vi "Process Data.vi"(7 "AdasLvTemplate in":refnum<class "AdasLvTemplate.lvclass">, 8 "error in":errorcluster, 11 "Node in":refnum<class "AMS Chiller Template.lvclass">) -> (0 "error out":errorcluster, 3 "Node out":refnum<class "AMS Chiller Template.lvclass">, 5 "AdasLvTemplate out":refnum<class "AdasLvTemplate.lvclass">)   [LabVIEW 2023, in "AMS Chiller Template.lvlib" / "AMS Chiller Template.lvclass"]
uses:
  AMS Chiller Template.lvclass
  <vilib>/ADAS Replay HIL/ADAS Plugin Utilities/AdasLvTemplate/AdasLvTemplate.lvclass
  AMS Chiller Template.lvclass/AMS Chiller Template.ctl
  C:/Program Files/National Instruments/AMS plugin/Capabilities/Capabilities/High Level Capabilities/Chiller/Control Mode Read Array.vi
  C:/Program Files/National Instruments/AMS plugin/Capabilities/Capabilities/High Level Capabilities/Chiller/Control Mode Write Array.vi
  C:/Program Files/National Instruments/AMS plugin/Capabilities/Capabilities/High Level Capabilities/Chiller/Output Enable Read Array.vi
  C:/Program Files/National Instruments/AMS plugin/Capabilities/Capabilities/High Level Capabilities/Chiller/Output Enable Write Array.vi
  C:/Program Files/National Instruments/AMS plugin/Capabilities/Capabilities/High Level Capabilities/Chiller/Temperature Min Read Array.vi
  C:/Program Files/National Instruments/AMS plugin/Capabilities/Capabilities/High Level Capabilities/Chiller/Temperature Max Read Array.vi
  C:/Program Files/National Instruments/AMS plugin/Capabilities/Capabilities/High Level Capabilities/Chiller/Temperature Grad Read Array.vi
  C:/Program Files/National Instruments/AMS plugin/Capabilities/Capabilities/High Level Capabilities/Chiller/Temperature Read Array.vi
  C:/Program Files/National Instruments/AMS plugin/Capabilities/Capabilities/High Level Capabilities/Chiller/Pressure Min Read Array.vi
  C:/Program Files/National Instruments/AMS plugin/Capabilities/Capabilities/High Level Capabilities/Chiller/Pressure Max Read Array.vi
  C:/Program Files/National Instruments/AMS plugin/Capabilities/Capabilities/High Level Capabilities/Chiller/Pressure Grad Read Array.vi
  C:/Program Files/National Instruments/AMS plugin/Capabilities/Capabilities/High Level Capabilities/Chiller/Pressure Read Array.vi
  C:/Program Files/National Instruments/AMS plugin/Capabilities/Capabilities/High Level Capabilities/Chiller/Flow Max Read Array.vi
  C:/Program Files/National Instruments/AMS plugin/Capabilities/Capabilities/High Level Capabilities/Chiller/Flow Min Read Array.vi
  C:/Program Files/National Instruments/AMS plugin/Capabilities/Capabilities/High Level Capabilities/Chiller/Flow Read Array.vi
  C:/Program Files/National Instruments/AMS plugin/Capabilities/Capabilities/High Level Capabilities/Chiller/Temperature Write Array.vi
  C:/Program Files/National Instruments/AMS plugin/Capabilities/Capabilities/High Level Capabilities/Chiller/Error Channels Write Array.vi
  C:/Program Files/National Instruments/AMS plugin/Capabilities/Capabilities/High Level Capabilities/Chiller/Pressure Write Array.vi
  C:/Program Files/National Instruments/AMS plugin/Capabilities/Capabilities/High Level Capabilities/Chiller/Flow Grad Read Array.vi
  C:/Program Files/National Instruments/AMS plugin/Capabilities/Capabilities/High Level Capabilities/Chiller/Flow Write Array.vi
  C:/Program Files/National Instruments/AMS plugin/Capabilities/Capabilities/High Level Capabilities/Chiller/Chiller.lvclass
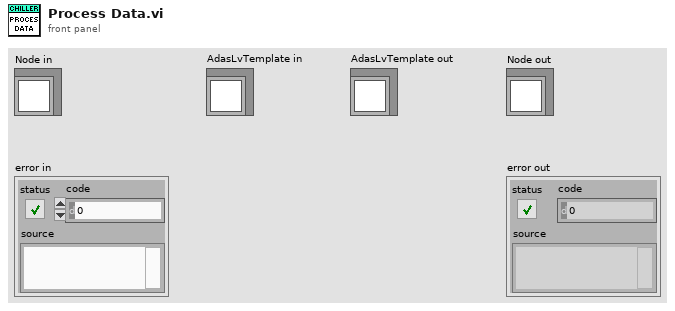
[diagram p1: front panel]
types:
  T1 = typedef "AMS Chiller Template.lvlib/AMS Chiller Template.lvclass/Configuration Params.ctl" = cluster{"Common":T2, "Amount of Channels":u32, "Address":string}
  T2 = typedef "Template Node.lvlib/Template Node.lvclass/Common Configuration Params.ctl" = cluster{"Iteration Interval (s)":dbl, "T0 (ns)":u64, "Priority":i32, "Processor":i32, "Wait in Ready State":bool}
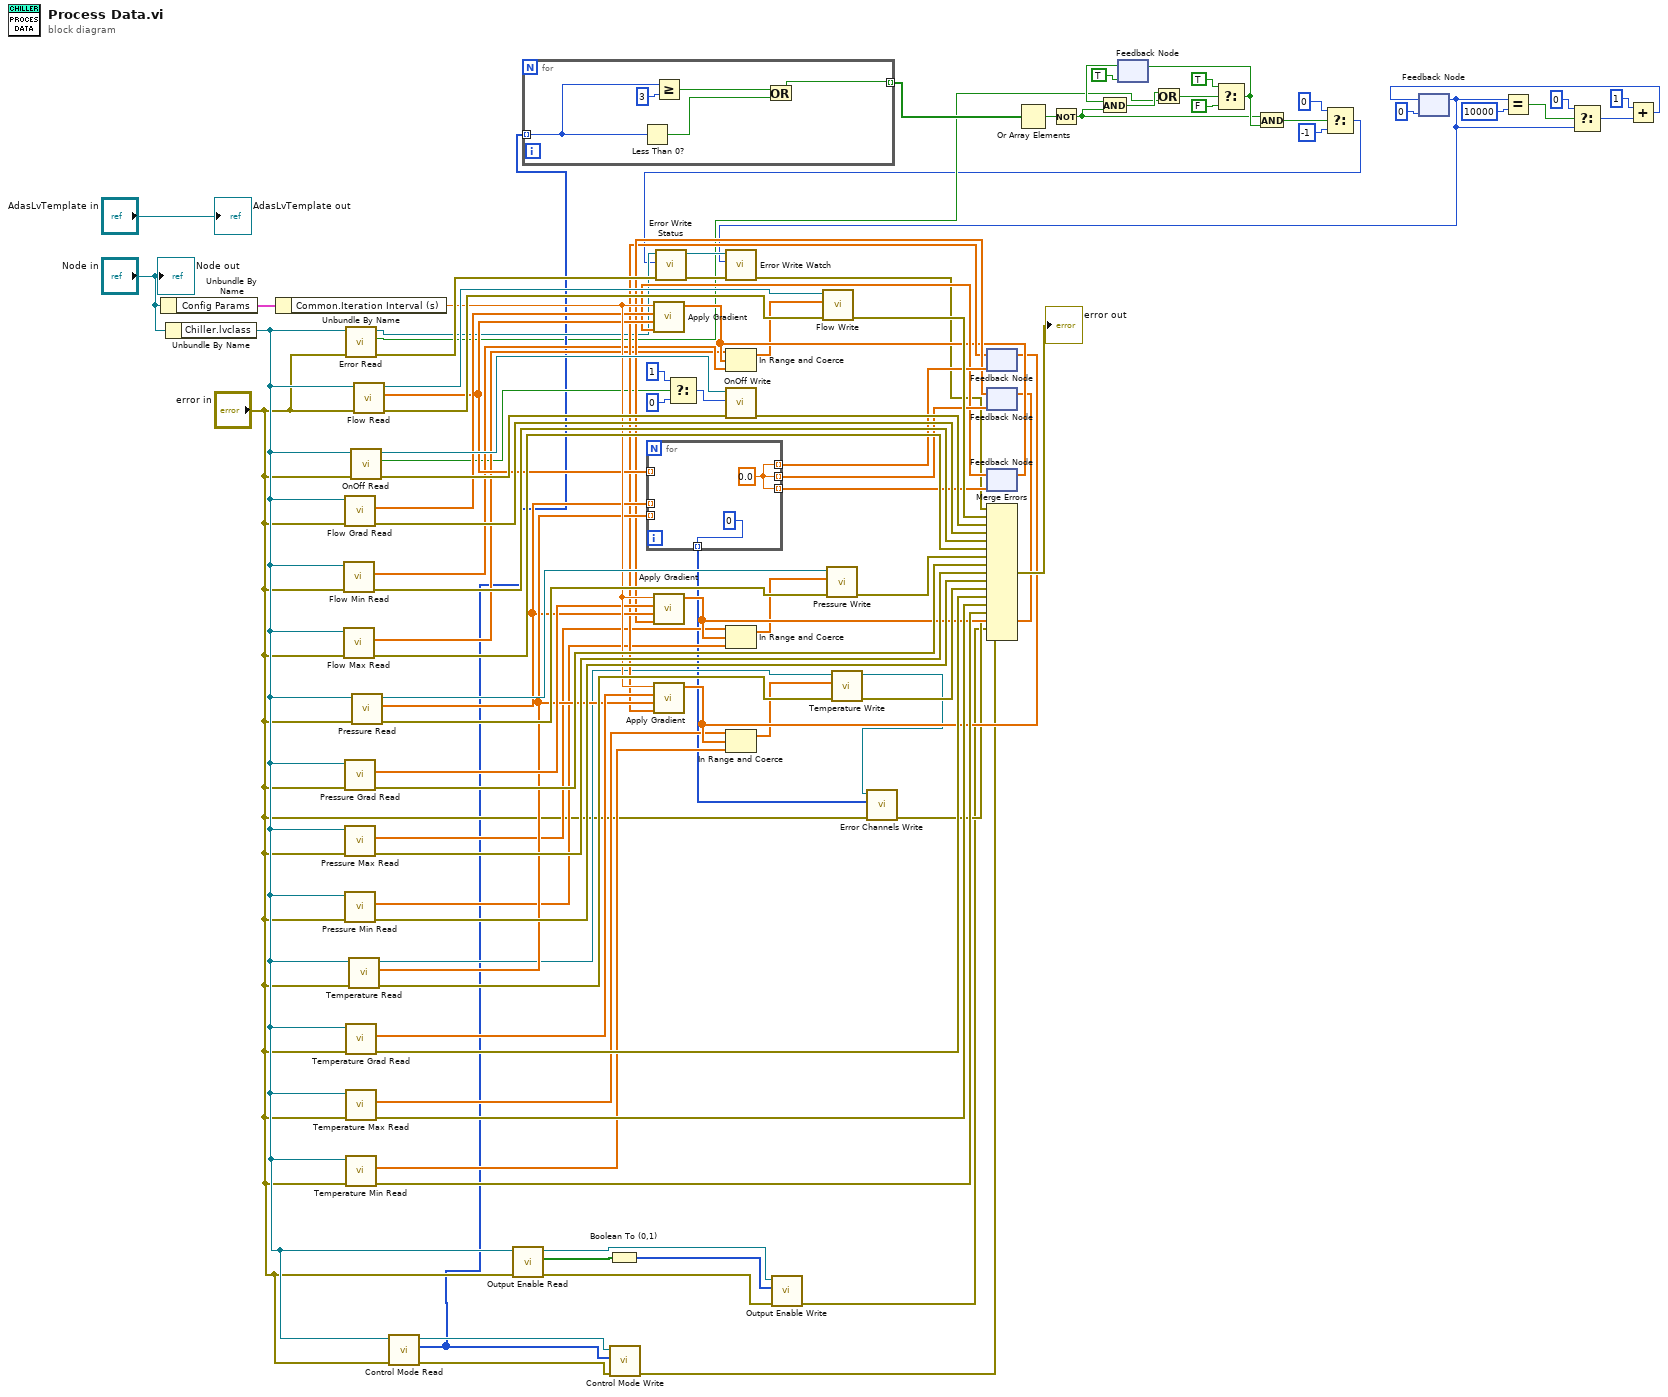
[diagram p0: block diagram]
diagram:
  n1 = Unbundle By Name("Node in") -> ("Config Params"=w71:T1)
  n2 = Unbundle By Name("Node in") -> ("Chiller.lvclass"=w26:refnum<class "Chiller.lvclass">)
  n3 = Unbundle By Name(w71) -> ("Common.Iteration Interval (s)"=w70:dbl)
  n4 = call-poly "Flow Min Read.vi"("error in"="error in", "Chiller in"=w26) -> ("error out"=w83:errorcluster, "Flow Min SP"=w56:dbl[])  [unwired: 6 in, 2 out]
  n5 = call-poly "Flow Max Read.vi"("error in"="error in", "Chiller in"=w26) -> ("error out"=w82:errorcluster, "Flow Max SP"=w55:dbl[])  [unwired: 6 in, 2 out]
  n6 = call-poly "Flow Grad Read.vi"("error in"="error in", "Chiller in"=w26) -> ("error out"=w84:errorcluster, "Flow SP"=w69:dbl[])  [unwired: 6 in, 2 out]
  n7 = call-poly "Pressure Grad Read.vi"("error in"="error in", "Chiller in"=w26) -> ("error out"=w80:errorcluster, "Pressure SP"=w68:dbl[])  [unwired: 6 in, 2 out]
  n8 = call-poly "Pressure Max Read.vi"("error in"="error in", "Chiller in"=w26) -> ("error out"=w79:errorcluster, "Pressure Max SP"=w51:dbl[])  [unwired: 6 in, 2 out]
  n9 = call-poly "Pressure Min Read.vi"("error in"="error in", "Chiller in"=w26) -> ("error out"=w78:errorcluster, "Pressure Min SP"=w50:dbl[])  [unwired: 6 in, 2 out]
  n10 = call "Error Read.vi"("error in"="error in", "Chiller in"=w26) -> ("error out"=w91:errorcluster, "Error ACT"=w3:bool, "Chiller out"=w41:refnum<class "Chiller.lvclass">)  [unwired: 6 in, 1 out]
  n11 = call-poly "Temperature Grad Read.vi"("error in"="error in", "Chiller in"=w26) -> ("error out"=w76:errorcluster, "Temperature SP"=w67:dbl[])  [unwired: 6 in, 2 out]
  n12 = call-poly "Temperature Max Read.vi"("error in"="error in", "Chiller in"=w26) -> ("error out"=w75:errorcluster, "Temperature Max SP"=w47:dbl[])  [unwired: 6 in, 2 out]
  n13 = call-poly "Temperature Min Read.vi"("error in"="error in", "Chiller in"=w26) -> ("error out"=w74:errorcluster, "Temperature Min SP"=w48:dbl[])  [unwired: 6 in, 2 out]
  n14 = call-poly "Temperature Read.vi"("error in"="error in", "Chiller in"=w26) -> ("error out"=w85:errorcluster, "Temperature SP"=w63:dbl[], "Chiller out"=w39:refnum<class "Chiller.lvclass">)  [unwired: 6 in, 1 out]
  n15 = call "OnOff Read.vi"("error in"="error in", "Chiller in"=w26) -> ("error out"=w89:errorcluster, "OnOff ACT"=w43:bool, "Chiller out"=w88:refnum<class "Chiller.lvclass">)  [unwired: 6 in, 1 out]
  n16 = call-poly "Pressure Read.vi"("error in"="error in", "Chiller in"=w26) -> ("error out"=w86:errorcluster, "Pressure SP"=w62:dbl[], "Chiller out"=w87:refnum<class "Chiller.lvclass">)  [unwired: 6 in, 1 out]
  n17 = call-poly "Flow Read.vi"("error in"="error in", "Chiller in"=w26) -> ("error out"=w93:errorcluster, "Flow SP"=w61:dbl[], "Chiller out"=w92:refnum<class "Chiller.lvclass">)  [unwired: 6 in, 1 out]
  n18 = call-poly "Control Mode Read.vi"("error in"="error in", "Chiller In"=w26) -> ("error out"=w28:errorcluster, "Control Mode CTL"=w24:u16[], "Chiller out"=w27:refnum<class "Chiller.lvclass">)  [unwired: 6 in, 1 out]
  n19 = call-poly "Output Enable Read.vi"("error in"="error in", "Chiller in"=w26) -> ("error out"=w31:errorcluster, "Output Enable ACT"=w34:bool[], "Chiller out"=w32:refnum<class "Chiller.lvclass">)  [unwired: 7 in]
  n20 = for {
    tunnel: w24 -> [w101] mode=indexing
    tunnel: [w97] -> w4 mode=indexing
    n21 = Less Than 0?(x=w101) -> (x < 0?=w99:bool)
    n22 = Greater Or Equal?(x=w101, y=u16 3) -> (x >= y?=w100:bool)
    n23 = Or(x=w100, y=w99) -> (x .or. y?=w97:bool)
  }
  n24 = Boolean To (0,1)(Boolean=w34) -> (0, 1=w33:i16[])
  n25 = call-poly "Control Mode Write.vi"("error in"=w28, "Control Mode STS"=w24, "Chiller In"=w27) -> ("error out"=w29:errorcluster)  [unwired: 7 in, 1 out]
  n26 = for {
    tunnel: [w103] -> w66 mode=indexing
    tunnel: [w103] -> w65 mode=indexing
    tunnel: w62 -> [_] mode=indexing
    tunnel: [w103] -> w64 mode=indexing
    tunnel: w63 -> [_] mode=indexing
    tunnel: w61 -> [_] mode=indexing
    tunnel: [0] -> w38 mode=indexing
    w103 = 0.0 ("Current Setpoint")
  }
  n27 = Select(t=1, s=w43, f=0) -> (s? t:f=w42:i32)
  n28 = call "OnOff Write.vi"("error in"=w89, "OnOff STS"=w42, "Chiller in"=w88) -> ("error out"=w96:errorcluster)  [unwired: 7 in, 1 out]
  n29 = call-poly "Output Enable Write.vi"("error in"=w31, "Output Enable STS"=w33, "Chiller in"=w32) -> ("error out"=w30:errorcluster)  [unwired: 7 in, 1 out]
  n30 = feedback #1(w64) -> (w58:dbl[])
  n31 = call "Apply Gradient.vi"("Reminder"=w58, "Setpoint"=w63, "Gradient"=w67, "Iteration Interval"=w70) -> ("Array"=w49:dbl[])  [unwired: 7 in]
  n32 = In Range and Coerce(upper limit=w47, x=w49, lower limit=w48) -> (coerced(x)=w46:dbl[])  [unwired: 1 out]
  n33 = call-poly "Temperature Write.vi"("error in"=w85, "Temperature AV"=w46, "Chiller in"=w39) -> ("error out"=w77:errorcluster, "Chiller out"=w37:refnum<class "Chiller.lvclass">)  [unwired: 7 in]
  n34 = call-poly "Error Channels Write.vi"("error in"="error in", "Error Channels STS"=w38, "Chiller in"=w37) -> ("error out"=w36:errorcluster)  [unwired: 7 in, 1 out]
  n35 = feedback-in #1(w49) -> ()
  n36 = feedback #2(w65) -> (w59:dbl[])
  n37 = call "Apply Gradient.vi"("Reminder"=w59, "Setpoint"=w62, "Gradient"=w68, "Iteration Interval"=w70) -> ("Array"=w53:dbl[])  [unwired: 7 in]
  n38 = In Range and Coerce(upper limit=w51, x=w53, lower limit=w50) -> (coerced(x)=w52:dbl[])  [unwired: 1 out]
  n39 = call-poly "Pressure Write.vi"("error in"=w86, "Pressure AV"=w52, "Chiller in"=w87) -> ("error out"=w81:errorcluster)  [unwired: 7 in, 1 out]
  n40 = feedback-in #2(w53) -> ()
  n41 = feedback #3(w66) -> (w60:dbl[])
  n42 = call "Apply Gradient.vi"("Reminder"=w60, "Setpoint"=w61, "Gradient"=w69, "Iteration Interval"=w70) -> ("Array"=w57:dbl[])  [unwired: 7 in]
  n43 = In Range and Coerce(upper limit=w55, x=w57, lower limit=w56) -> (coerced(x)=w54:dbl[])  [unwired: 1 out]
  n44 = call-poly "Flow Write.vi"("error in"=w93, "Flow AV"=w54, "Chiller in"=w92) -> ("error out"=w73:errorcluster)  [unwired: 7 in, 1 out]
  n45 = feedback-in #3(w57) -> ()
  n46 = Or Array Elements(Boolean array=w4) -> (logical OR=w14:bool)
  n47 = Not(x=w14) -> (.not. x?=w8:bool)
  n48 = feedback #4(TRUE) -> (w9:bool)
  n49 = And(x=w9, y=w8) -> (x .and. y?=w7:bool)
  n50 = Or(x=w7, y=w3) -> (x .or. y?=w13:bool)
  n51 = Select(t=TRUE, s=w13, f=FALSE) -> (s? t:f=w10:bool)
  n52 = feedback-in #4(w10) -> ()
  n53 = And(x=w8, y=w10) -> (x .and. y?=w6:bool)
  n54 = Select(t=0, s=w6, f=-1) -> (s? t:f=w2:i32)
  n55 = call "Error Write Status.vi"("error in"=w91, "Error STS"=w2, "Chiller in"=w41) -> ("error out"=w90:errorcluster, "Chiller out"=w40:refnum<class "Chiller.lvclass">)  [unwired: 7 in]
  n56 = feedback #5(0) -> (w1:i32)
  n57 = call "Error Write Watch.vi"("error in"=w90, "Watchdog STS"=w1, "Chiller in"=w40) -> ("error out"=w35:errorcluster)  [unwired: 7 in, 1 out]
  n58 = Merge Errors(w35, w73, w96, w84, w83, w82, w81, w80, w79, w78, w77, w76, w75, w74, w36, w30, w29) -> (→"error out":errorcluster)
  n59 = Equal?(x=w1, y=10000) -> (x = y?=w19:bool)
  n60 = Select(t=0, s=w19, f=w1) -> (s? t:f=w18:i32)
  n61 = Add(x=1, y=w18) -> (x+y=w23:i32)
  n62 = feedback-in #5(w23) -> ()
  "Node out" <- "Node in"
  "AdasLvTemplate out" <- "AdasLvTemplate in"
